vi "Format Client Request (Internal).vi"(8 "error in (no error)":errorcluster, 9 "params":variant, 10 "method":string) -> (0 "error out":errorcluster, 3 "JSON Value out":variant)   [LabVIEW 2020, in "JSON-RPC Lib.lvlib" / "JSONRPC Client.lvclass"]
uses:
  JSONRPC Client.lvclass
  Variant Data Manipulation/Insert Element at Start.vi
  Variant Data Manipulation/Variant Data Manipulation.lvlib
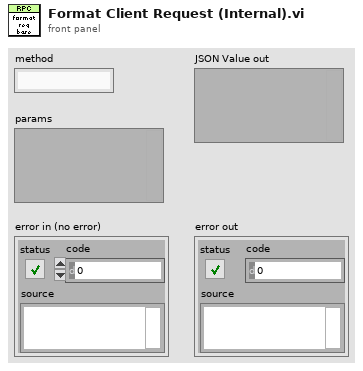
[diagram p1: front panel]
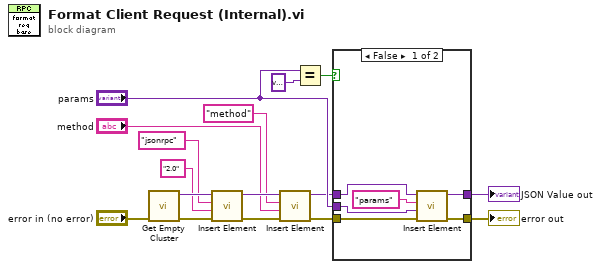
[diagram p0: block diagram]
diagram:
  n1 = call "Get Empty Cluster.vi"("error in (no error)"="error in (no error)") -> ("error out"=w9:errorcluster, "Variant (Cluster) out"=w8:variant)  [unwired: 9 in]
  n2 = call-poly "Insert Element.vi"("error in (no error)"=w9, "element"="2.0" ("String"), "Name"="jsonrpc", "Variant (Cluster) in"=w8) -> ("error out"=w10:errorcluster, "Variant (Cluster) out"=w7:variant)  [unwired: 6 in]
  n3 = call-poly "Insert Element.vi"("error in (no error)"=w10, "element"="method", "Name"="method", "Variant (Cluster) in"=w7) -> ("error out"=w11:errorcluster, "Variant (Cluster) out"=w12:variant)  [unwired: 6 in]
  n4 = Equal?(x="params", y=variant) -> (x = y?=w16:bool)
  n5 = case shown="False" w16 {
    tunnel: w11 -> [w22 w23]
    tunnel: w12 -> [w19 w24]
    tunnel: [w21 w24] -> w6
    tunnel: [w20 w23] -> w14
    tunnel: "params" -> [w17 _]
    frame False {
      n6 = call-poly "Insert Element.vi"("error in (no error)"=w22, "element"=w17, "Name"="params", "Variant (Cluster) in"=w19) -> ("error out"=w20:errorcluster, "Variant (Cluster) out"=w21:variant)  [unwired: 6 in]
    }
    frame True {
    }
  }
  "error out" <- w14
  "JSON Value out" <- w6
